vi "Log String.vi"(5 "Level":T1, 6 "String":string, 8 "error in (no error)":errorcluster, 11 "Asynchronous Application Log in":refnum<class "Asynchronous Application Log.lvclass">) -> (0 "error out":errorcluster, 3 "Asynchronous Application Log out":refnum<class "Asynchronous Application Log.lvclass">)   [LabVIEW 2016, in "Stream Log.lvlib" / "Asynchronous Application Log.lvclass"]
doc: "--\nCopyright © 2017 Composed SystemsI All rights reserved.\n\nAuthor: Jon McBee <jon.mcbee@composed.io>\n\nThis library is provided \"AS IS\" ,WITHOUT WARRANTIES OR\nCONDITIONS OF ANY KIND, either express or implied.\n\nComposed Systems -- composed.io\n\nStream 0.0.1.1\nJon McBee - Composed Systems\nCopyright (c) 2017, Composed Systems"
uses:
  <userlib>/Composed Systems/Stream/Log/Asynchronous Application Log/Asynchronous Application Log.lvclass
  C:/Program Files (x86)/National Instruments/LabVIEW 2016/user.lib/Composed Systems/Stream/Log/Application Log/Application Log.lvclass
  <userlib>/Composed Systems/Stream/Log/Application Log/Log Level.ctl
  <userlib>/Composed Systems/Stream/Log/Asynchronous Application Log/Message.ctl
  <userlib>/Composed Systems/Stream/Log/Asynchronous Application Log/Entry Type.ctl
  <userlib>/Composed Systems/Stream/Log/Log Sink/Log Sink.lvclass
  <userlib>/Composed Systems/Stream/Log/Asynchronous Application Log/Asynchronous Application Log.lvclass/Asynchronous Application Log.ctl
  <userlib>/Composed Systems/Stream/Log/Application Log/Application Log.lvclass
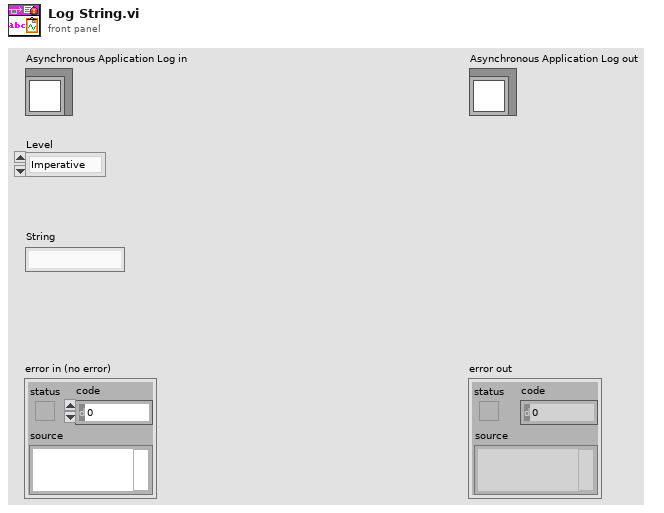
[diagram p1: front panel]
types:
  T1 = typedef "Stream Log.lvlib/Application Log.lvclass/Log Level.ctl" = enum16{"Imperative", "Major", "Minor", "Debug", "Off"}
  T2 = typedef "Stream Log.lvlib/Asynchronous Application Log.lvclass/Entry Type.ctl" = enum16{"Kill Worker", "Log Entry"}
  T3 = typedef "Stream Log.lvlib/Asynchronous Application Log.lvclass/Message.ctl" = cluster{"Entry Type":T2, "String":string, "Sinks":refnum<data-value>[], "Parallel Sinks?":bool}
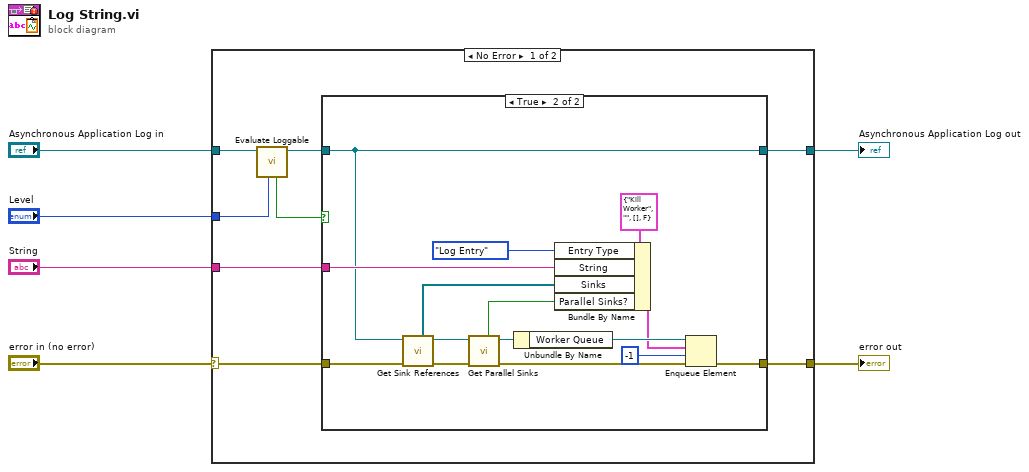
[diagram p0: block diagram]
diagram:
  n1 = case shown="No Error" "error in (no error)" {
    selector: "error in (no error)" -> [w10 w32]
    tunnel: [w7 w32] -> w5
    tunnel: "Asynchronous Application Log in" -> [w14 w33]
    tunnel: [w8 w33] -> w3
    tunnel: "Level" -> [w13 _]
    tunnel: "String" -> [w11 _]
    frame No Error {
      n2 = call <userlib>:"Evaluate Loggable.vi"("Level"=w13, "Application Log in"=w14) -> ("Application Log out"=w9:refnum<class "Asynchronous Application Log.lvclass">, "Log?"=w12:bool)  [unwired: 8 in]
      n3 = case shown="True" w12 {
        tunnel: w11 -> [_ w25]
        tunnel: w10 -> [w15 w31]
        tunnel: w9 -> [w16 w20]
        tunnel: [w16 w20] -> w8
        tunnel: [w15 w18] -> w7
        frame False {
        }
        frame True {
          n4 = call <userlib>:"Get Sink References.vi"("error in (no error)"=w31, "Application Log in"=w20) -> ("error out"=w30:errorcluster, "Application Log out"=w29:refnum<class "Asynchronous Application Log.lvclass">, "Sinks"=w26:refnum<data-value>[])  [unwired: 6 in, 1 out]
          n5 = call <userlib>:"Get Parallel Sinks.vi"("error in (no error)"=w30, "Application Log in"=w29) -> ("error out"=w23:errorcluster, "Application Log out"=w22:refnum<class "Asynchronous Application Log.lvclass">, "Parallel Sinks"=w27:bool)  [unwired: 7 in]
          n6 = Unbundle By Name(w22) -> ("Worker Queue"=w21:refnum<queue>)
          n7 = Bundle By Name(cluster=T3 {"Entry Type"=enum."Kill Worker", "String"="", "Sinks"=[], "Parallel Sinks?"=FALSE} ("Message"), "Entry Type"=Entry_Type."Log Entry", "String"=w25, "Sinks"=w26, "Parallel Sinks?"=w27) -> (w19:T3)
          n8 = Enqueue Element(queue=w21, element=w19, timeout in ms (-1)=-1, error in (no error)=w23) -> (error out=w18:errorcluster)  [unwired: 2 out]
        }
      }
    }
    frame Error {
    }
  }
  "error out" <- w5
  "Asynchronous Application Log out" <- w3
